vi "Config Continuous Interval.vi"(8 "error in":errorcluster, 10 "Interval (0)":dbl min=0.0 max=99999999.0 step=0.1 format="%#_10f", 11 "VISA resource name":refnum<visa-resource-name>) -> (0 "error out":errorcluster, 3 "VISA resource name out":refnum<visa-resource-name>)   [LabVIEW 2019, in "Andeen-Hagerling 2700(400 firmware).lvlib"]
doc: "Sets the measurement rate for continuous mode measurements by setting the minimum time from one measurement to the next."
uses:
  Andeen-Hagerling 2700(400 firmware).lvlib
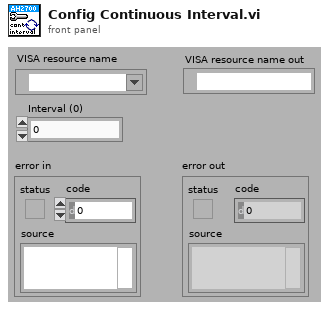
[diagram p1: front panel]
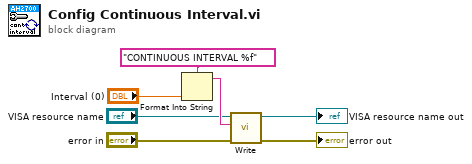
[diagram p0: block diagram]
diagram:
  n1 = Format Into String(format string="CONTINUOUS INTERVAL %f", "Interval (0)") -> (resulting string=w6:string)  [unwired: 2 in, 1 out]
  n2 = call "Write.vi"("error in"="error in", "command"=w6, "VISA resource name"="VISA resource name") -> ("error out"=→"error out":errorcluster, "VISA resource name out"=→"VISA resource name out":refnum<visa-resource-name>)  [unwired: 7 in]
